vi "GetDatetime String.vi"(10 "error in (no error)":errorcluster, 11 "u?":i32) -> (1 "error out":errorcluster, 2 "Datetime DBL":dbl, 3 "date/time string":string, 4 "date/time string 3":string, 5 "date/time string 2":string, 7 "D. M. Y":string)   [LabVIEW 2021]
doc: "Get Datetime string\njiangsong@outlook.com\nSina: @sushu1051\n2016-08-25 13:28:30"
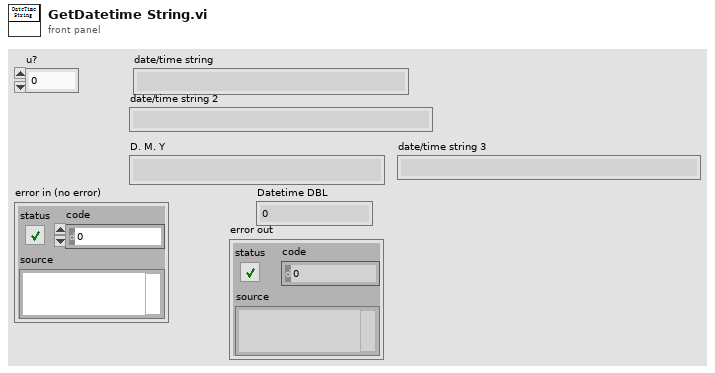
[diagram p1: front panel]
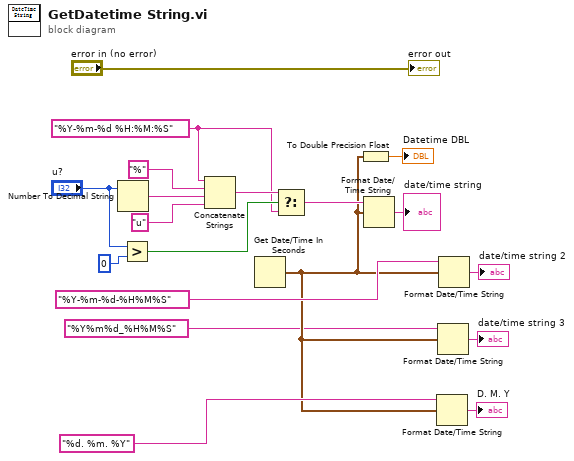
[diagram p0: block diagram]
diagram:
  w12 = "%Y-%m-%d %H:%M:%S" ("time format string (%c)")
  n1 = Number To Decimal String(number="u?") -> (decimal integer string=w17:string)  [unwired: 1 in]
  n2 = Greater?(x="u?", y=0) -> (0:w14:bool)
  n3 = Concatenate Strings(w12, "%" ("string"), w17, "u" ("string")) -> (w13:string)
  n4 = Get Date/Time In Seconds() -> (seconds since 1Jan1904=w3:timestamp)
  n5 = Select(t=w13, s=w14, f=w12) -> (s? t:f=w11:string)
  n6 = To Double Precision Float(number=w3) -> (double precision float=→"Datetime DBL":dbl)
  n7 = Format Date/Time String(time format string (%c)=w11, seconds (now)=w3) -> (date/time string=→"date/time string":string)  [unwired: 1 in]
  n8 = Format Date/Time String(time format string (%c)="%d. %m. %Y", seconds (now)=w3) -> (date/time string=→"D. M. Y":string)  [unwired: 1 in]
  n9 = Format Date/Time String(time format string (%c)="%Y%m%d_%H%M%S", seconds (now)=w3) -> (date/time string=→"date/time string 3":string)  [unwired: 1 in]
  n10 = Format Date/Time String(time format string (%c)="%Y-%m-%d-%H%M%S", seconds (now)=w3) -> (date/time string=→"date/time string 2":string)  [unwired: 1 in]
  "error out" <- "error in (no error)"
